vi "remove scheduled message.vi"(10 "Scheduled messages in":T1[](array[typedef]), 11 "scheduled message":T1) -> (3 "Scheduled messages out":T1[](array[typedef]))   [LabVIEW 2018, in "Message scheduler.lvlib"]
uses:
  Message Scheduler/Message scheduler.lvlib
  Type Defs/scheduled message cluster.ctl
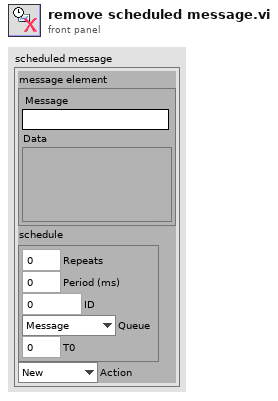
[diagram p1: front panel]
types:
  T1 = typedef "Message scheduler.lvlib/scheduled message cluster.ctl" = cluster{"message element":cluster{"Message":string, "Data":variant}, "schedule":cluster{"Repeats":i16, "Period (ms)":u32, "ID":u32, "Queue":enum16{"Message", "Comms"}, "T0":u32}, "Action":enum16{"New", "Remove", "Quit"}}
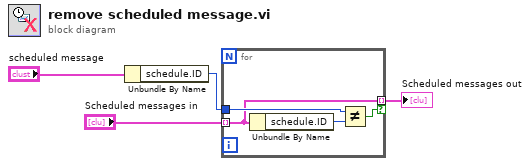
[diagram p0: block diagram]
diagram:
  n1 = Unbundle By Name("scheduled message") -> ("schedule.ID"=w1:u32)
  n2 = for {
    tunnel: "Scheduled messages in" -> [w7] mode=indexing
    tunnel: [w7] -> w3 mode=indexing if=w5
    tunnel: w1 -> [w8]
    n3 = Unbundle By Name(w7) -> ("schedule.ID"=w6:u32)
    n4 = Not Equal?(x=w8, y=w6) -> (x != y?=w5:bool)
  }
  "Scheduled messages out" <- w3
